vi "4_Sum1toN.vi"() -> ()   [LabVIEW 2015]
panel:
  out "Sum of 1 to N":u32
  in  "Enter a number":u32
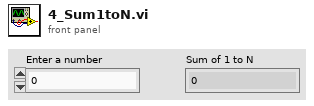
[diagram p1: front panel]
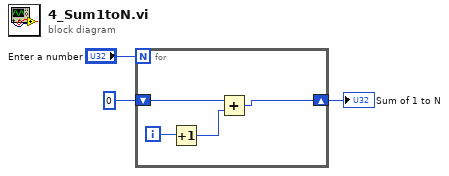
[diagram p0: block diagram]
diagram:
  n1 = for {
    N: "Enter a number" -> [_]
    shift-right: [w4] -> w1
    shift-left: 0 -> [w6]
    i -> [w7]
    n2 = Increment(x=w7) -> (x+1=w5:i32)
    n3 = Add(x=w6, y=w5) -> (x+y=w4:i32)
  }
  "Sum of 1 to N" <- w1
